vi "string_to_array.vi"(1 "string":string) -> (0 "array":string[](array[string]))   [LabVIEW 2012]
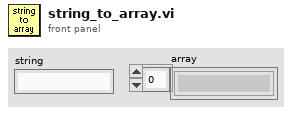
[diagram p1: front panel]
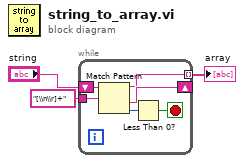
[diagram p0: block diagram]
diagram:
  n1 = while {
    tunnel: "[\\n\\r]+" ("regular expression") -> [w8]
    shift-right: [w7] -> _
    shift-left: "string" -> [w9]
    tunnel: [w6] -> w2 mode=indexing
    stop <- w4 stop-if-true
    n2 = Match Pattern(string=w9, regular expression=w8) -> (before substring=w6:string, after substring=w7:string, offset past match=w5:i32)  [unwired: 1 in, 1 out]
    n3 = Less Than 0?(x=w5) -> (x < 0?=w4:bool)
  }
  "array" <- w2
